vi "QueryServer_GetTestDataTypesParameters.vi"(6 "error in (no error)":errorcluster, 9 "gRPCid":T2) -> (0 "error out":errorcluster, 2 "TestDataTypesParameters":T1, 3 "gRPCid out":T2)   [LabVIEW 2019, in "labview-grpc-query-server.lvlib"]
uses:
  labview-grpc-query-server.lvlib
  QueryServer_gRPCid.ctl
  QueryServer_TestDataTypesParameters.ctl
  build/Debug/labview_grpc_server.dll
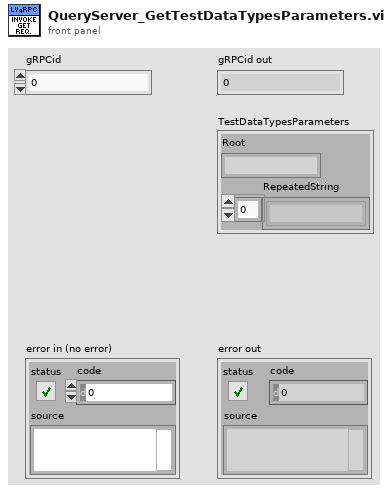
[diagram p1: front panel]
types:
  T1 = typedef "labview-grpc-query-server.lvlib/QueryServer_TestDataTypesParameters.ctl" = cluster{"Root":string, "RepeatedString":string[]}
  T2 = typedef "labview-grpc-query-server.lvlib/QueryServer_gRPCid.ctl" = u64
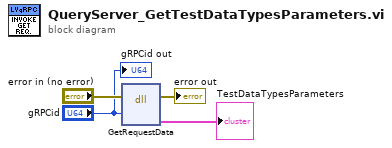
[diagram p0: block diagram]
diagram:
  n1 = dll-call lib="C:/dev/labview-grpc-server/build/Debug/labview_grpc_server.dll" fn="GetRequestData"(error in="error in (no error)", "id"="gRPCid") -> (error out=→"error out":errorcluster, "TestDataTypesParameters"=→"TestDataTypesParameters":T1)  [unwired: 5 in, 1 out]
  "gRPCid out" <- "gRPCid"
